vi "DAQ_1CH.vi"(3 "error in (no error)":errorcluster) -> (10 "error out":errorcluster)   [LabVIEW 2014]
uses:
  set_get.ctl
  CMD DAQ enum.ctl
  patiant and daq params.ctl
  <vilib>/DAQmx/create/channels.llb/DAQmx Create Channel (AI-Voltage-Basic).vi
  <vilib>/DAQmx/configure/timing.llb/DAQmx Timing (Sample Clock).vi
  <vilib>/DAQmx/read.llb/DAQmx Read (Analog 1D DBL 1Chan NSamp).vi
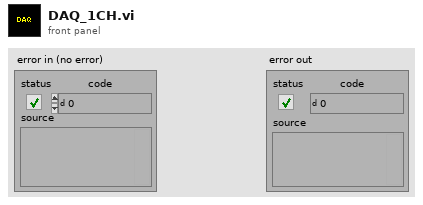
[diagram p1: front panel]
types:
  T1 = typedef "set_get.ctl" = enum16{"Set", "Get"}
  T2 = cluster{"CMD UI":refnum<queue>, "CMD REP":refnum<queue>, "CMD DA":refnum<queue>, "CMD DAQ":refnum<queue>, "CMD LOG":refnum<queue>, "Data LOG":refnum<queue>, "Data Display":refnum<queue>}
  T3 = typedef "patiant and daq params.ctl" = cluster{"DAQ Parameters":cluster{"Sampling rate":dbl, "Max_volt":dbl, "Min_volt":dbl, "DAQmx Physical Channels \nHR,SC":tag, "Resting State":bool}, "Patient Info":cluster{"Patient Name":string, "Patient ID":string, "Patient Age":dbl, "Gender":string}}
  T4 = typedef "CMD DAQ enum.ctl" = enum16{"Init DAQ", "Init Read From File", "DAQ", "Read From File", "Stop DAQ", "Stop Read From File", "Exit"}
  T5 = enum16{"open", "replace", "create", "open or create", "replace or create", "replace or create with confirmation"}
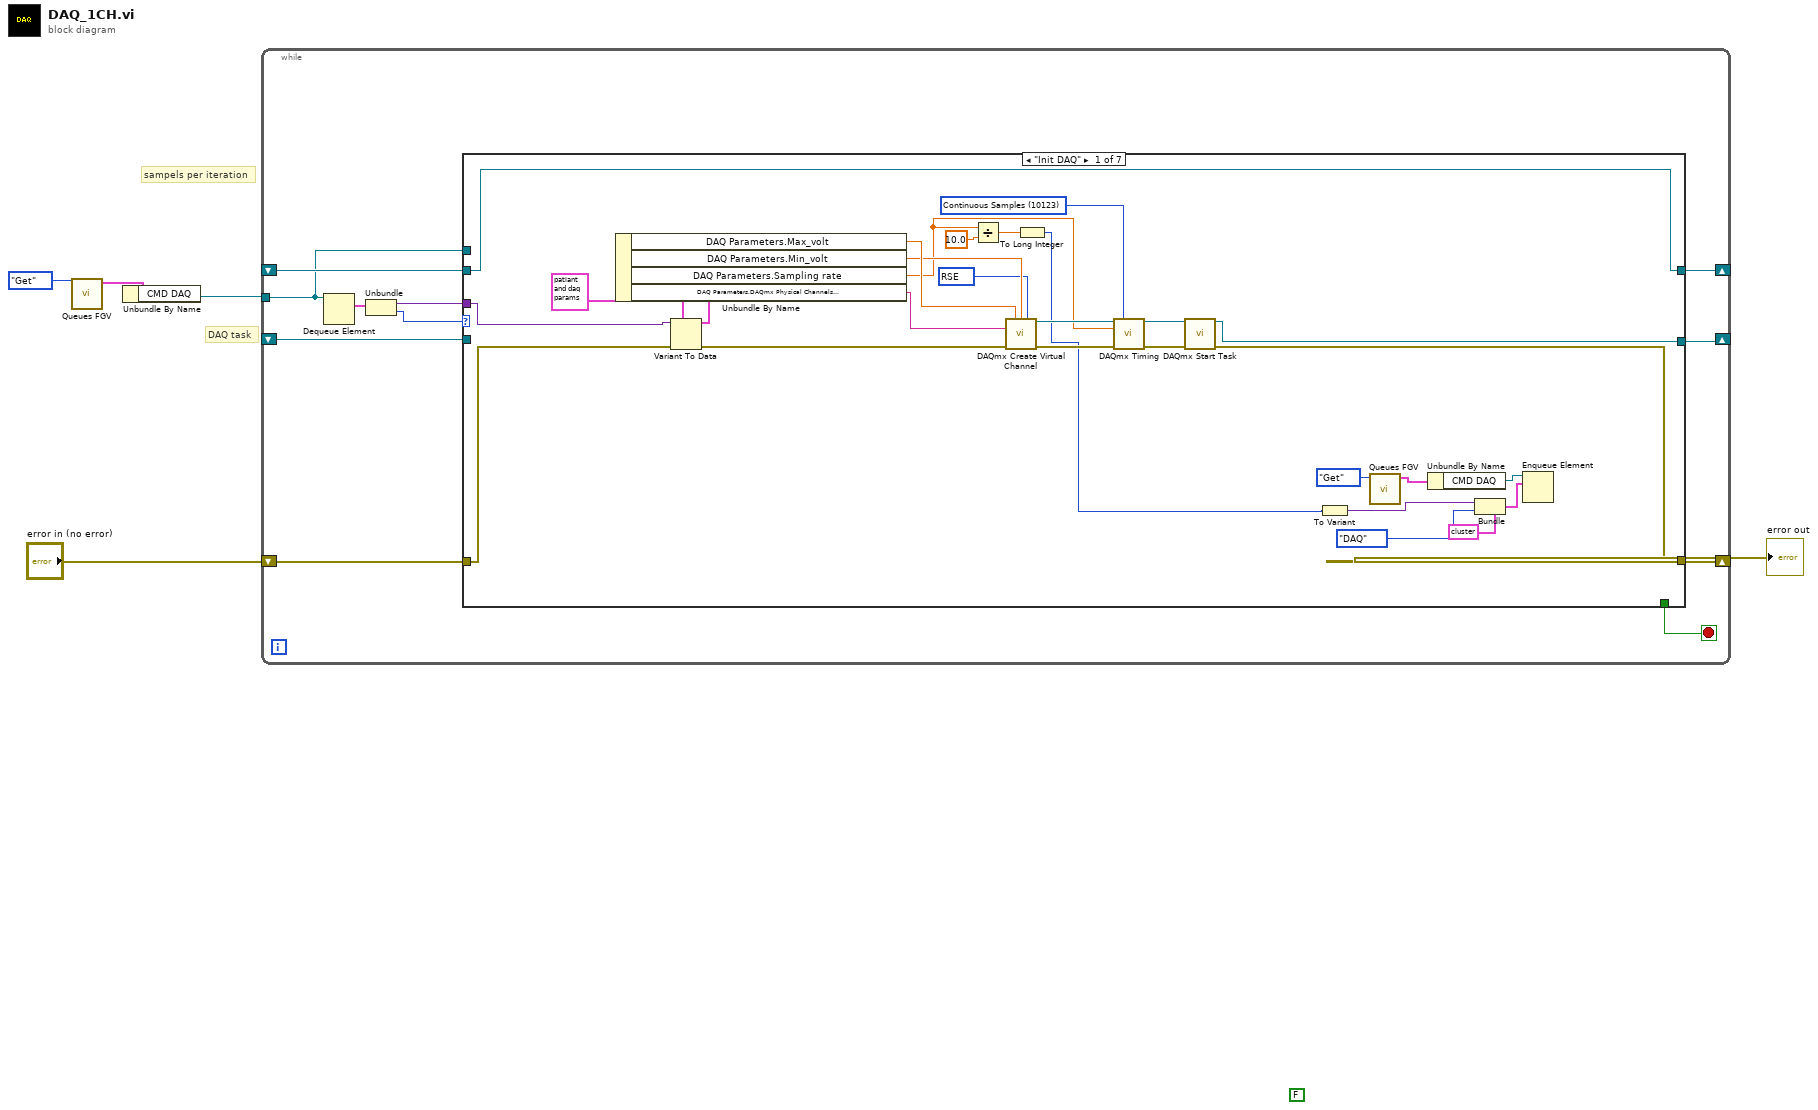
[diagram p0: block diagram]
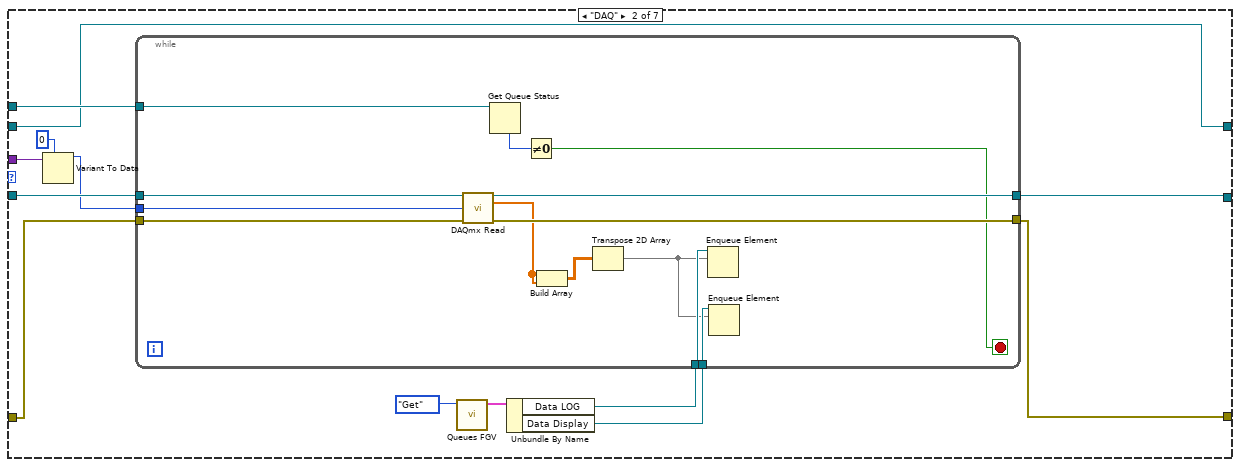
[diagram p2: hidden frame]
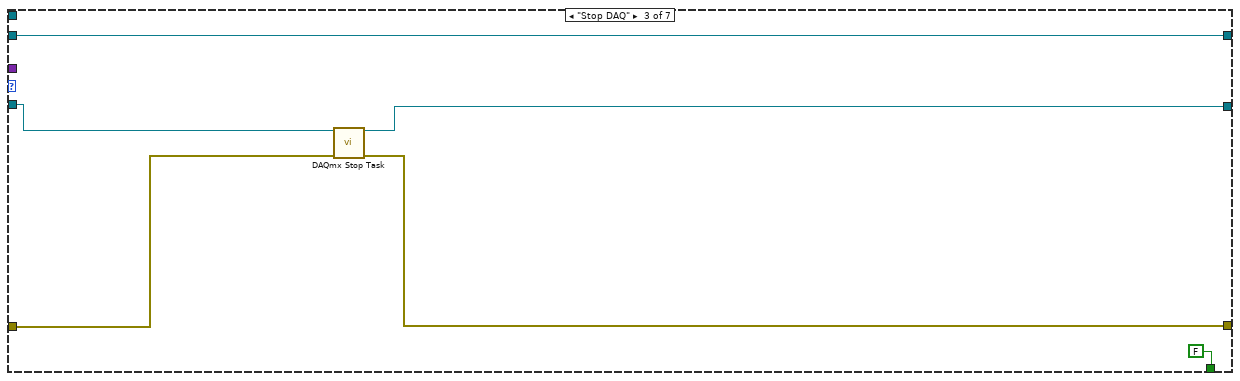
[diagram p3: hidden frame]
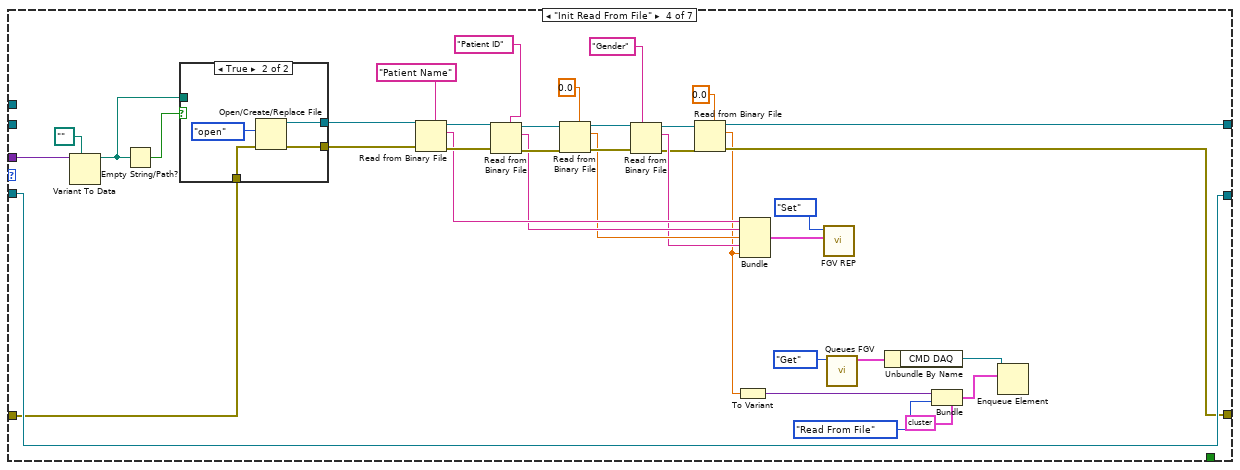
[diagram p4: hidden frame]
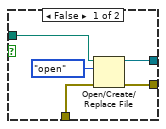
[diagram p5: hidden frame]
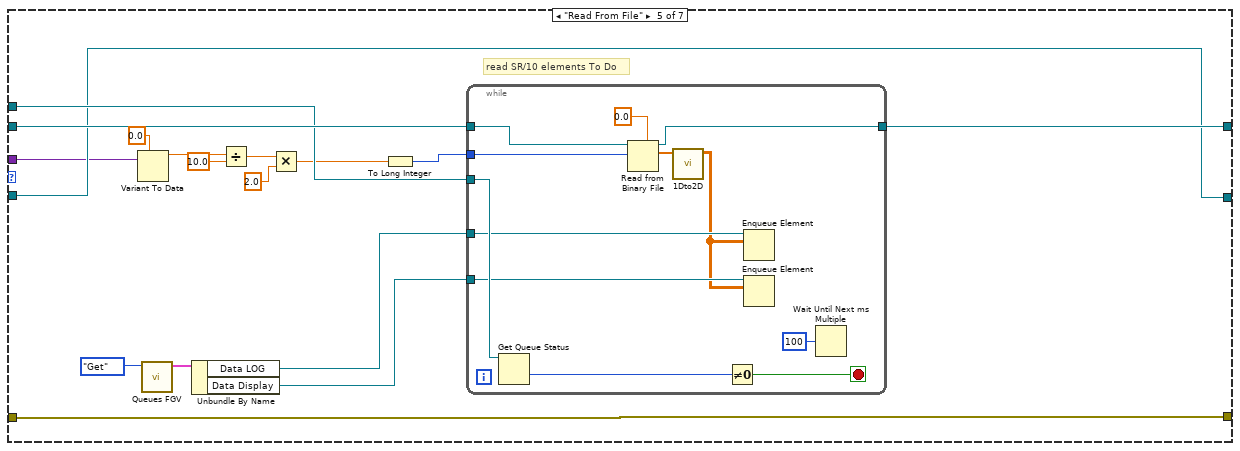
[diagram p6: hidden frame]
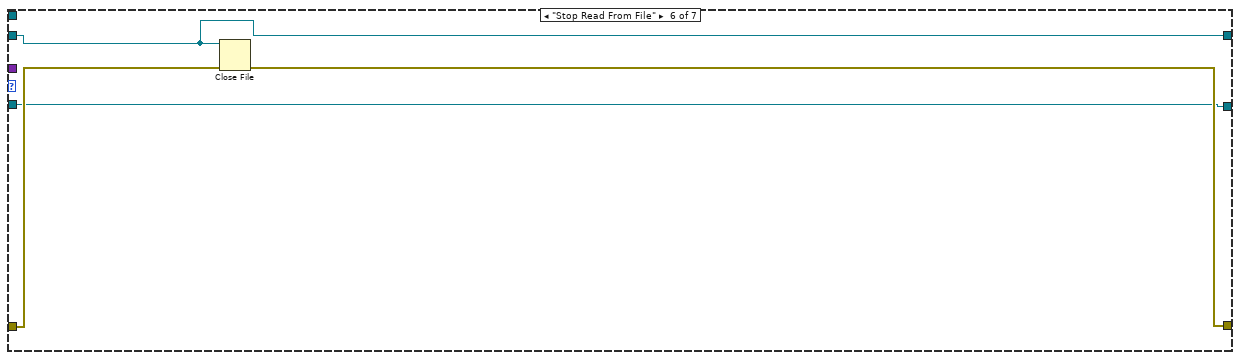
[diagram p7: hidden frame]
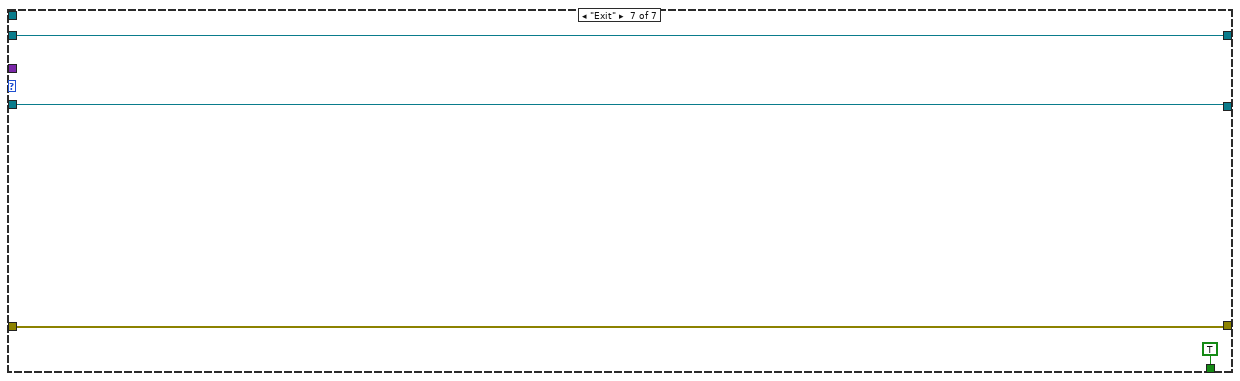
[diagram p8: hidden frame]
diagram:
  (unwired) FALSE
  # "DAQ task"
  # "sampels per iteration"
  n1 = call "Queues FGV.vi"("Enum"=set_get."Get") -> ("Queues"=w4:T2)  [unwired: 10 in]
  n2 = Unbundle By Name(w4) -> ("CMD DAQ"=w3:refnum<queue>)
  n3 = while {
    tunnel: w3 -> [w6]
    shift-right: [w13] -> w2
    shift-left: "error in (no error)" -> [w14]
    shift-right: [w11] -> _
    shift-left: _ -> [w10]
    shift-right: [w8] -> _
    shift-left: _ -> [w7]
    stop <- w12 stop-if-true
    n4 = Dequeue Element(queue=w6) -> (element=w16:cluster{variant, T4})  [unwired: 2 in, 3 out]
    n5 = Unbundle(w16) -> (w9:variant, w15:T4)
    n6 = case shown="\"Init DAQ\"" w15 {
      tunnel: [_ _ FALSE ("Boolean 2") _ _ _ TRUE ("Boolean 2")] -> w12
      tunnel: w14 -> [w32 w56 w76 w86 w132 w154 w156]
      tunnel: [w28 w55 w75 w85 w132 w153 w156] -> w13
      tunnel: [w27 w54 w74 w113 w131 w152 w158] -> w11
      tunnel: w10 -> [_ w57 w72 w113 w131 w152 w158]
      tunnel: w9 -> [w30 w49 _ w112 w130 _ _]
      tunnel: [w18 w50 w71 w87 w138 w155 w159] -> w8
      tunnel: w7 -> [w18 w50 w71 _ w139 w155 w159]
      tunnel: w6 -> [_ w51 _ _ w137 _ _]
      frame "Init DAQ" {
        w37 = 10083 items=["default"=-1, "RSE"=10083, "NRSE"=10078, "Differential"=10106, "Pseudodifferential"=12529] ("input terminal configuration")
        w42 = 10123 items=["Finite Samples"=10178, "Continuous Samples"=10123, "Hardware Timed Single Point"=12522] ("sample mode")
        n7 = Variant To Data(error in=w32, type=T3 {"DAQ Parameters"={"Sampling rate"=0.0, "Max_volt"=0.0, "Min_volt"=0.0, "DAQmx Physical Channels \nHR,SC"="", "Resting State"=FALSE}, "Patient Info"={"Patient Name"="", "Patient ID"="", "Patient Age"=0.0, "Gender"=""}} ("output cluster"), Variant=w30) -> (data=w41:T3, error out=w31:errorcluster)
        n8 = Unbundle By Name(w41) -> ("DAQ Parameters.Max_volt"=w39:dbl, "DAQ Parameters.Min_volt"=w38:dbl, "DAQ Parameters.Sampling rate"=w29:dbl, "DAQ Parameters.DAQmx Physical Channels \nHR,SC"=w40:tag)
        n9 = Divide(x=w29, y=10.0) -> (x/y=w33:dbl)
        n10 = call-poly <vilib>:"DAQmx Create Virtual Channel.vi"("maximum value"=w39, "minimum value"=w38, "input terminal configuration"=w37, "physical channels"=w40, "error in"=w31) -> ("task out"=w44:refnum<k21>, "error out"=w43:errorcluster)  [unwired: 9 in]
        n11 = To Long Integer(number=w33) -> (32bit integer=w19:i32)
        n12 = call-poly <vilib>:"DAQmx Timing.vi"("task/channels in"=w44, "sample mode"=w42, "rate"=w29, "error in"=w43) -> ("task out"=w36:refnum<k21>, "error out"=w35:errorcluster)  [unwired: 10 in]
        n13 = call <vilib>:"DAQmx Start Task.vi"("task/channels in"=w36, "error in"=w35) -> ("task out"=w27:refnum<k21>, "error out"=w28:errorcluster)  [unwired: 12 in]
        n14 = To Variant(anything=w19) -> (Variant=w20:variant)
        n15 = call "Queues FGV.vi"("Enum"=set_get."Get") -> ("Queues"=w22:T2)  [unwired: 10 in]
        n16 = Unbundle By Name(w22) -> ("CMD DAQ"=w23:refnum<queue>)
        n17 = Bundle(cluster=cluster{variant, T4} {variant, enum."Init DAQ"}, w20, CMD_DAQ_enum."DAQ") -> (w26:cluster{variant, T4})
        n18 = Enqueue Element(queue=w23, element=w26) -> ()  [unwired: 2 in, 3 out]
      }
      frame "DAQ" {
        n19 = Variant To Data(type=0, Variant=w49) -> (data=w47:i32)  [unwired: 1 in, 1 out]
        n20 = call "Queues FGV.vi"("Enum"=set_get."Get") -> ("Queues"=w52:T2)  [unwired: 10 in]
        n21 = Unbundle By Name(w52) -> ("Data LOG"=w46:refnum<queue>, "Data Display"=w45:refnum<queue>)
        n22 = while {
          tunnel: [w70] -> w55
          tunnel: [w69] -> w54
          tunnel: w57 -> [w62]
          tunnel: w56 -> [w60]
          tunnel: w51 -> [w66]
          tunnel: w47 -> [w61]
          tunnel: w46 -> [w65]
          tunnel: w45 -> [w64]
          stop <- w67 stop-if-true
          n23 = call-poly <vilib>:"DAQmx Read.vi"("task/channels in"=w62, "number of samples per channel"=w61, "error in"=w60) -> ("task out"=w69:refnum<k21>, "data"=w58:dbl[], "error out"=w70:errorcluster)  [unwired: 10 in]
          n24 = Get Queue Status(queue=w66) -> (# elements in queue=w68:i32)  [unwired: 2 in, 7 out]
          n25 = Not Equal To 0?(x=w68) -> (x != 0?=w67:bool)
          n26 = Build Array(w58, w58) -> (w59:dbl[][])
          n27 = Transpose 2D Array(2D array=w59) -> (transposed array=w63:dbl[][])
          n28 = Enqueue Element(queue=w65, element=w63) -> ()  [unwired: 2 in, 3 out]
          n29 = Enqueue Element(queue=w64, element=w63) -> ()  [unwired: 2 in, 3 out]
        }
      }
      frame "Stop DAQ" {
        n30 = call <vilib>:"DAQmx Stop Task.vi"("task/channels in"=w72, "error in"=w76) -> ("task out"=w74:refnum<k21>, "error out"=w75:errorcluster)  [unwired: 12 in]
      }
      frame "Init Read From File" {
        n31 = Variant To Data(type=path "", Variant=w112) -> (data=w109:path)  [unwired: 1 in, 1 out]
        n32 = Empty String/Path?(string/path=w109) -> (empty?=w110:bool)
        n33 = case shown="True" w110 {
          tunnel: w109 -> [w117 _]
          tunnel: [w116 w121] -> w108
          tunnel: [w115 w120] -> w107
          tunnel: w86 -> [w114 w119]
          frame False {
            n34 = Open/Create/Replace File(file path (use dialog)=w117, error in=w114, operation (0:open)=T5."open") -> (refnum out=w116:refnum<file>, error out=w115:errorcluster)  [unwired: 3 in, 1 out]
          }
          frame True {
            n35 = Open/Create/Replace File(error in=w119, operation (0:open)=T5."open") -> (refnum out=w121:refnum<file>, error out=w120:errorcluster)  [unwired: 4 in, 1 out]
          }
        }
        n36 = Read from Binary File(5:"Patient Name", 8:w107, 11:w108) -> (0:w105:errorcluster, 2:w96:string, 3:w104:refnum<file>)  [unwired: 3 in, 1 out]
        n37 = Read from Binary File(5:"Patient ID", 8:w105, 11:w104) -> (0:w103:errorcluster, 2:w95:string, 3:w101:refnum<file>)  [unwired: 3 in, 1 out]
        n38 = Read from Binary File(5:0.0, 8:w103, 11:w101) -> (0:w102:errorcluster, 2:w94:dbl, 3:w100:refnum<file>)  [unwired: 3 in, 1 out]
        n39 = Read from Binary File(7:"Gender", 8:w102, 11:w100) -> (0:w90:errorcluster, 2:w93:string, 3:w89:refnum<file>)  [unwired: 3 in, 1 out]
        n40 = Read from Binary File(5:0.0, 8:w90, 11:w89) -> (0:w85:errorcluster, 2:w79:dbl, 3:w87:refnum<file>)  [unwired: 3 in, 1 out]
        n41 = To Variant(anything=w79) -> (Variant=w80:variant)
        n42 = Bundle(w96, w95, w94, w93, w79) -> (w78:cluster{string, string, dbl, string, dbl})  [unwired: 1 in]
        n43 = call "FGV REP.vi"("Patient Info"=w78, "Enum"=set_get."Set") -> ()  [unwired: 9 in, 1 out]
        n44 = call "Queues FGV.vi"("Enum"=set_get."Get") -> ("Queues"=w91:T2)  [unwired: 10 in]
        n45 = Unbundle By Name(w91) -> ("CMD DAQ"=w84:refnum<queue>)
        n46 = Bundle(cluster=cluster{variant, T4} {variant, enum."Init DAQ"}, w80, CMD_DAQ_enum."Read From File") -> (w81:cluster{variant, T4})
        n47 = Enqueue Element(queue=w84, element=w81) -> ()  [unwired: 2 in, 3 out]
      }
      frame "Read From File" {
        # "read SR/10 elements To Do"
        n48 = Variant To Data(type=0.0, Variant=w130) -> (data=w129:dbl)  [unwired: 1 in, 1 out]
        n49 = call "Queues FGV.vi"("Enum"=set_get."Get") -> ("Queues"=w136:T2)  [unwired: 10 in]
        n50 = Unbundle By Name(w136) -> ("Data LOG"=w134:refnum<queue>, "Data Display"=w133:refnum<queue>)
        n51 = Divide(x=w129, y=10.0) -> (x/y=w127:dbl)
        n52 = Multiply(x=w127, y=2.0) -> (x*y=w125:dbl)
        n53 = To Long Integer(number=w125) -> (32bit integer=w124:i32)
        n54 = while {
          tunnel: w139 -> [w151]
          tunnel: [w150] -> w138
          tunnel: w137 -> [w147]
          tunnel: w134 -> [w146]
          tunnel: w133 -> [w145]
          tunnel: w124 -> [w143]
          stop <- w148 stop-if-true
          n55 = Get Queue Status(queue=w147) -> (# elements in queue=w149:i32)  [unwired: 2 in, 7 out]
          n56 = Read from Binary File(5:0.0, 10:w143, 11:w151) -> (2:w141:dbl[], 3:w150:refnum<file>)  [unwired: 3 in, 2 out]
          n57 = call "1Dto2D.vi"("Array"=w141) -> ("output array"=w140:dbl[][])  [unwired: 10 in]
          n58 = Not Equal To 0?(x=w149) -> (x != 0?=w148:bool)
          n59 = Enqueue Element(queue=w146, element=w140) -> ()  [unwired: 2 in, 3 out]
          n60 = Enqueue Element(queue=w145, element=w140) -> ()  [unwired: 2 in, 3 out]
          n61 = Wait Until Next ms Multiple(millisecond multiple=u32 100) -> ()  [unwired: 1 out]
        }
      }
      frame "Stop Read From File" {
        n62 = Close File(refnum=w155, error in=w154) -> (error out=w153:errorcluster)  [unwired: 1 out]
      }
      frame "Exit" {
      }
    }
  }
  "error out" <- w2
